vi "Pfeiffer Vacuum Digiline Relay Switch Point.vi"(8 "error in (no error)":errorcluster, 9 "DigiLine-Cluster":T1={"Parameter"=0, "Parameter\nread only<->describe"=FALSE, "Pressure switch point (mbar)"=1.0} {"Pressure switch point (mbar)" min=5e-10 max=2000.0 step=1.0 format="%_3e"; "Parameter" items=[" Pressure switch point 1 [mbar]", " Pressure switch point 2 [mbar]"]}, 10 "Adress of unit":u16=1 min=1 max=999 step=1, 11 "VISA session in":refnum<visa-resource-name>) -> (0 "error out":errorcluster, 3 "response (data)":string)   [LabVIEW 2021]
doc: "This VI is an example of how to use the Pfeiffer Vacuum subVIs programmatically. This VI first initializes the instrument, takes measurements, then closes the instrument."
uses:
  <instrlib>/Pfeiffer Vacuum/Public/DigiLine/PV Digiline relay switch point - Cluster.ctl
  <instrlib>/Pfeiffer Vacuum/Pfeiffer Vacuum.lvlib
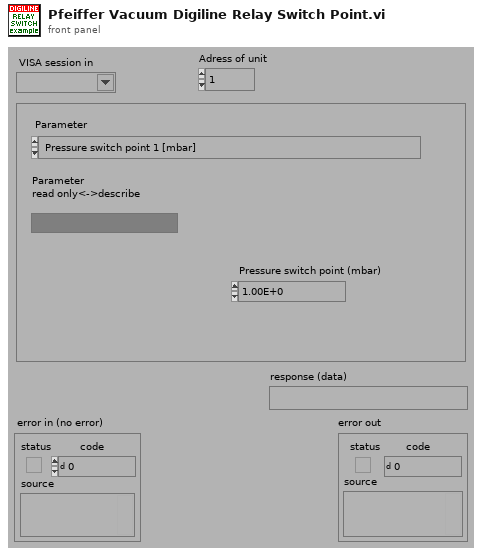
[diagram p1: front panel]
types:
  T1 = typedef "Pfeiffer Vacuum.lvlib/PV Digiline relay switch point - Cluster.ctl" = cluster{"Parameter":u16, "Parameter\nread only<->describe":bool, "Pressure switch point (mbar)":dbl}
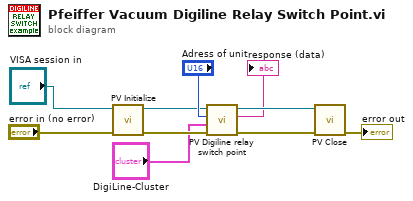
[diagram p0: block diagram]
diagram:
  n1 = call <instrlib>:"PV Initialize.vi"("error in (no error)"="error in (no error)", "VISA session in"="VISA session in") -> ("error out"=w4:errorcluster, "VISA session out"=w3:refnum<visa-resource-name>)  [unwired: 8 in]
  n2 = call <instrlib>:"PV Digiline relay switch point.vi"("error in (no error)"=w4, "DigiLine-Cluster"="DigiLine-Cluster", "Adress of unit"="Adress of unit", "VISA session"=w3) -> ("error out"=w10:errorcluster, "response (data)"=→"response (data)":string, "dup VISA session"=w9:refnum<visa-resource-name>)  [unwired: 5 in]
  n3 = call <instrlib>:"PV Close.vi"("VISA session"=w9, "error in (no error)"=w10) -> ("error out"=→"error out":errorcluster)  [unwired: 13 in]
